vi "validate_inputs.vi"(0 "chatcompletion_llm_interface in":refnum<class "llm_openai_chatmodels.lvclass">, 11 "error in (no error)":errorcluster) -> (4 "chatcompletion_llm_interface out":refnum<class "llm_openai_chatmodels.lvclass">, 15 "error out":errorcluster)   [LabVIEW 2020, in "llm_openai_chatmodels.lvclass"]
uses:
  llm_openai_chatmodels.lvclass
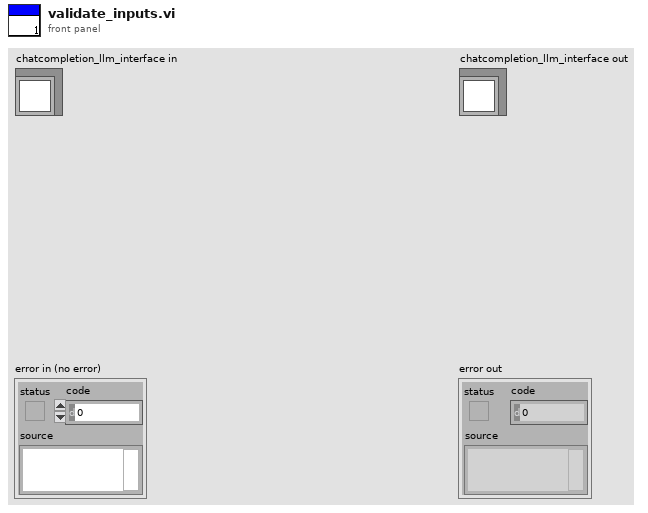
[diagram p1: front panel]
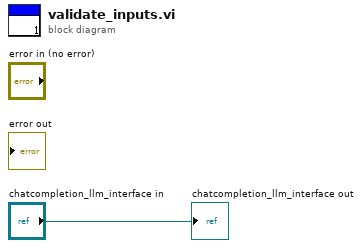
[diagram p0: block diagram]
diagram:
  "chatcompletion_llm_interface out" <- "chatcompletion_llm_interface in"
